vi "GetAppOutput.vi"(8 "error in (no error)":errorcluster, 11 "ModelValidation in":refnum<class "ModelValidationPlugin.lvclass">) -> (0 "error out":errorcluster, 3 "ModelValidation out":refnum<class "ModelValidationPlugin.lvclass">)   [LabVIEW 2017, in "AppPlugins.lvlib" / "ModelValidationPlugin.lvclass"]
uses:
  ModelValidationPlugin.lvclass
  C:/dev/Work/PARTF/Modules/AppPlugins/AppPluginBaseClass/AppPluginsBase.lvclass
  TypeDef/Output.ctl
  AppPluginBaseClass/AppPluginsBase.lvclass/AppPluginsBase.ctl
  ModelValidationPlugin.lvclass/ModelValidationPlugin.ctl
  AppPluginBaseClass/Accessors/Read clEvtReportArray.vi
  Accessors/Read ModelValidationConfig.vi
panel:
  out "Kalman gain":dbl[][](array[numeric])
  out "xk":dbl[][](array[numeric])
  out "Pk":dbl[][](array[numeric])
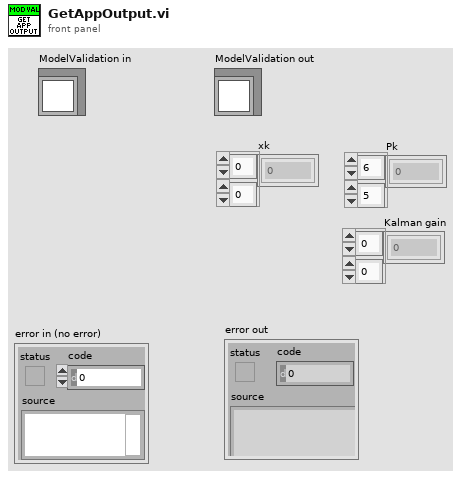
[diagram p1: front panel]
types:
  T1 = typedef "AppPlugins.lvlib/ModelValidationPlugin.lvclass/Output.ctl" = cluster{"xk":dbl[][], "Pk":dbl[][], "KalmanGain":dbl[][], "delta_t":dbl}
  T2 = typedef "EventPlugins.lvlib/EventPluginBaseClass.lvclass/clEvtReportArray.ctl" = T3[]
  T3 = typedef "EventPlugins.lvlib/EventPluginBaseClass.lvclass/clEvtReport.ctl" = cluster{"Timestamp":dbl, "Synx":cdb[], "Freq":dbl, "ROCOF":dbl, "ID":i16}
  T4 = typedef "AppPlugins.lvlib/ModelValidationPlugin.lvclass/Config.ctl" = cluster{"NoiseVariance":dbl, "Iindex":i32, "OffsetTime":dbl, "InterpolationFactor":i32, "Initial condition":cluster{"H0":dbl, "xd0":dbl, "D0":dbl}}
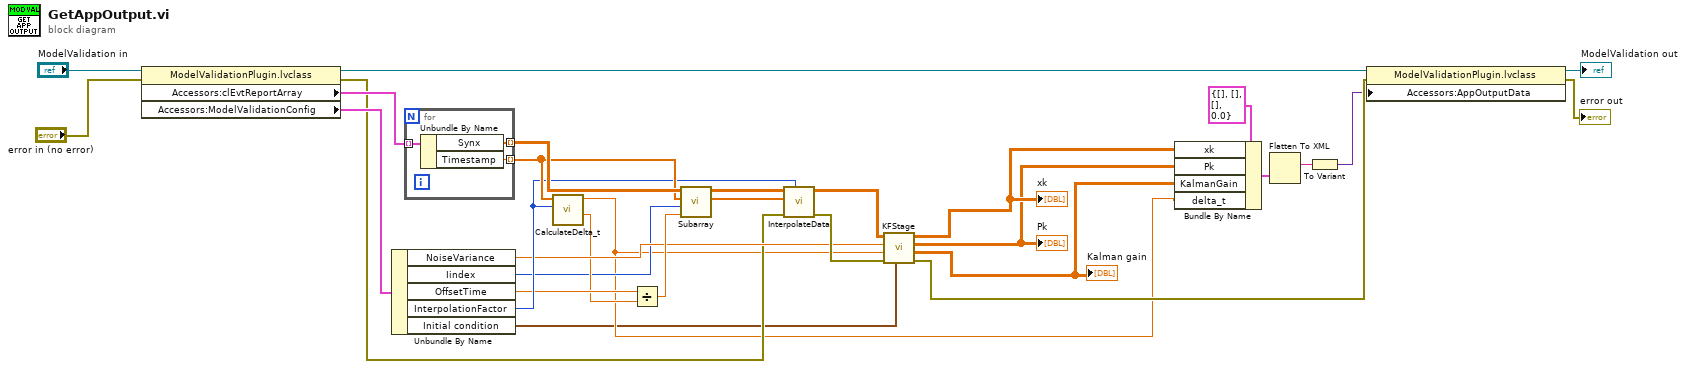
[diagram p0: block diagram]
diagram:
  n1 = property class="ModelValidationPlugin.lvclass"(reference="ModelValidation in", error in="error in (no error)") -> (reference out=w23:refnum<class "ModelValidationPlugin.lvclass">, error out=w3:errorcluster, "Accessors:clEvtReportArray"=w30:T2, "Accessors:ModelValidationConfig"=w10:T4)
  n2 = Unbundle By Name(w10) -> ("NoiseVariance"=w6:dbl, "Iindex"=w4:i32, "OffsetTime"=w8:dbl, "InterpolationFactor"=w9:i32, "Initial condition"=w1:cluster{"H0":dbl, "xd0":dbl, "D0":dbl})
  n3 = for {
    tunnel: [w33] -> w14 mode=indexing
    tunnel: w30 -> [w32] mode=indexing
    tunnel: [w31] -> w11 mode=indexing
    n4 = Unbundle By Name(w32) -> ("Synx"=w33:cdb[], "Timestamp"=w31:dbl)
  }
  n5 = call "CalculateDelta_t.vi"("InterpFactor"=w9, "Array"=w11) -> ("Reporting Rate"=w5:dbl, "delta_t"=w2:dbl)  [unwired: 8 in]
  n6 = Divide(x=w8, y=w5) -> (x/y=w7:dbl)
  n7 = call "Subarray.vi"("SamplesOffset"=w7, "I index"=w4, "Time"=w11, "Synx"=w14) -> ("Time subarray"=w12:dbl[], "Data subarray"=w13:cdb[][])  [unwired: 6 in]
  n8 = call "InterpolateData.vi"("Interp. factor"=w9, "error in (no error)"=w3, "Time"=w12, "Array"=w13) -> ("error out"=w16:errorcluster, "Array interpolated"=w15:cdb[][])  [unwired: 6 in]
  n9 = call "KFStage.vi"("Initial condition"=w1, "error in (no error)"=w16, "delta_t"=w2, "NoiseVariance"=w6, "Synx"=w15) -> ("error out"=w20:errorcluster, "KalmanGain"=w24:dbl[][], "Pk"=w25:dbl[][], "xk"=w26:dbl[][])  [unwired: 3 in]
  "Pk" <- w25
  "xk" <- w26
  "Kalman gain" <- w24
  n10 = Bundle By Name(cluster=T1 {"xk"=[], "Pk"=[], "KalmanGain"=[], "delta_t"=0.0} ("ModelValidationOutput"), "xk"=w26, "Pk"=w25, "KalmanGain"=w24, "delta_t"=w2) -> (w18:T1)
  n11 = Flatten To XML(anything=w18) -> (xml string=w19:string)
  n12 = To Variant(anything=w19) -> (Variant=w17:variant)
  n13 = property class="ModelValidationPlugin.lvclass"(reference=w23, error in=w20, "Accessors:AppOutputData"=w17) -> (reference out=→"ModelValidation out":refnum<class "ModelValidationPlugin.lvclass">, error out=→"error out":errorcluster)
